vi "Configure Input Control Model.vi"(8 "error in (no error)":errorcluster, 10 "Model":string(combo), 11 "VISA resource name":refnum<visa-resource-name>) -> (0 "error out":errorcluster, 3 "VISA resource name out":refnum<visa-resource-name>)   [LabVIEW 2015, in "IT8900A-E.lvlib"]
doc: "This command determines whether the input adjustment mode is controlled by the list value or by the FUNCtion command.\n:FIXed the regulating MODE is determined by the FUNCtion and MODE command.\n:LIST control mode is determined by the active LIST."
uses:
  <instrlib>/IT8900/IT8900A-E.lvlib
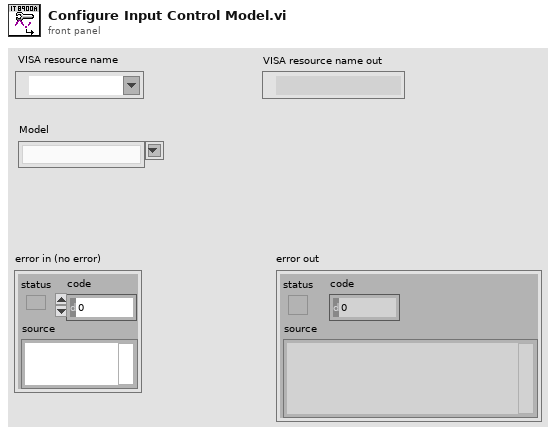
[diagram p1: front panel]
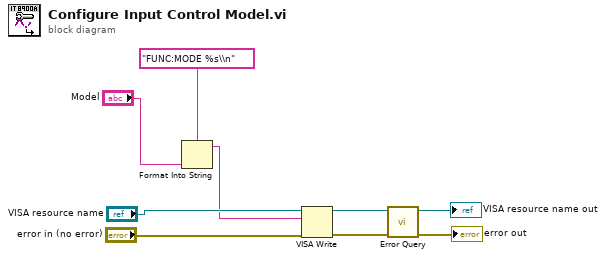
[diagram p0: block diagram]
diagram:
  n1 = Format Into String(format string="FUNC:MODE %s\\n", "Model") -> (resulting string=w1:string)  [unwired: 2 in, 1 out]
  n2 = VISA Write(VISA resource name="VISA resource name", write buffer=w1, error in (no error)="error in (no error)") -> (VISA resource name out=w4:refnum<visa-resource-name>, error out=w5:errorcluster)  [unwired: 1 out]
  n3 = call <instrlib>:"Error Query.vi"("error in (no error)"=w5, "VISA resource name"=w4) -> ("error out"=→"error out":errorcluster, "VISA resource name out"=→"VISA resource name out":refnum<visa-resource-name>)  [unwired: 6 in, 2 out]
